vi "FirstByte to ControlPacket.vi"(7 "MQTTVersion_50":refnum<class "MQTTVersion50.lvclass">, 11 "Packet First Byte":u8 format="%08b") -> (3 "Packet Type":refnum<class "ControlPacket.lvclass">)   [LabVIEW 2013, in "MQTT_Control_Packets_50.lvlib" / "MQTTVersion50.lvclass"]
uses:
  MQTTVersion50.lvclass
  ControlPacket/ControlPacket.lvclass
  AUTH/AUTH.lvclass
  ControlPacket/ControlPacket.lvclass/ControlPacket.ctl
  MQTT_311/MQTTVersion.lvclass
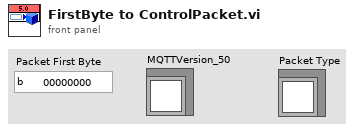
[diagram p1: front panel]
types:
  T1 = typedef "MQTT_Control_Packets.lvlib/ControlPacket.lvclass/Control Packet Type -- enum.ctl" = enum16{"Reserved", "CONNECT", "CONNACK", "PUBLISH", "PUBACK", "PUBREC", "PUBREL", "PUBCOMP", "SUBSCRIBE", "SUBACK", "UNSUBSCRIBE", "UNSUBACK", "PINGREQ", "PINGRESP", "DISCONNECT", "AUTH"}
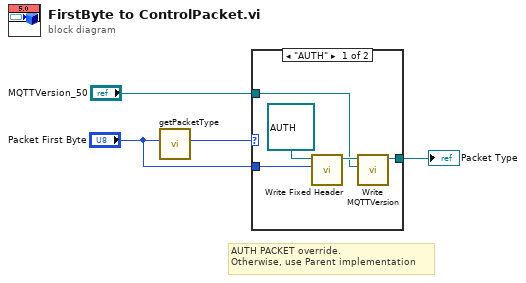
[diagram p0: block diagram]
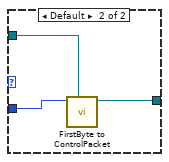
[diagram p2: hidden frame]
diagram:
  # "AUTH PACKET override.\nOtherwise, use Parent implementation"
  n1 = call "getPacketType.vi"("Packet First Byte"="Packet First Byte") -> ("Control Packet Type"=w4:T1)  [unwired: 10 in]
  n2 = case shown="\"AUTH\"" w4 {
    tunnel: "Packet First Byte" -> [w8 w12]
    tunnel: [w6 w11] -> w2
    tunnel: "MQTTVersion_50" -> [w5 w10]
    frame "AUTH" {
      n3 = call "Write Fixed Header.vi"("Fixed Header"=w8, "ControlPacket in"=refnum<class "AUTH.lvclass"> refnum ("MQTT_Control_Packets_50.lvlib:AUTH.lvclass")) -> ("ControlPacket out"=w7:refnum<class "AUTH.lvclass">)  [unwired: 9 in]
      n4 = call "Write MQTTVersion.vi"("MQTTVersion"=w5, "ControlPacket in"=w7) -> ("ControlPacket out"=w6:refnum<class "AUTH.lvclass">)  [unwired: 9 in]
    }
    frame Default {
      n5 = call-parent "FirstByte to ControlPacket.vi"("MQTTVersion"=w10, "Packet First Byte"=w12) -> ("Packet Type"=w11:refnum<class "ControlPacket.lvclass">)  [unwired: 9 in]
    }
  }
  "Packet Type" <- w2
